vi "State Change Core.vi"(8 "error in":errorcluster, 10 "Transition State":refnum<class "State Pattern.lvclass">, 11 "State in":refnum<class "State Pattern.lvclass">) -> (0 "error out":errorcluster, 3 "State out":refnum<class "State Pattern.lvclass">)   [LabVIEW 2021, in "State Pattern.lvclass"]
uses:
  State Pattern.lvclass
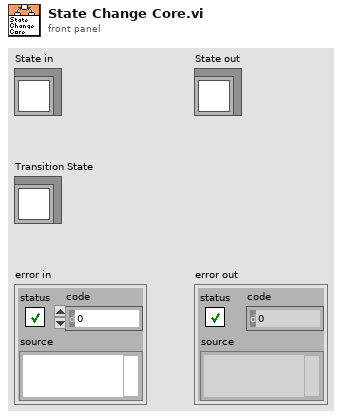
[diagram p1: front panel]
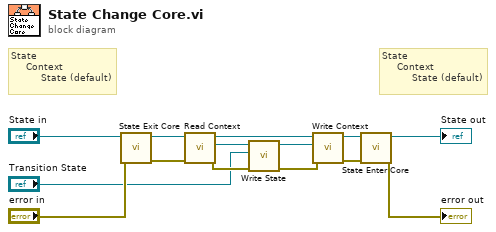
[diagram p0: block diagram]
diagram:
  # "State\n     Context\n          State (default)"
  # "State\n     Context\n          State (default)"
  n1 = call-dynamic "State Exit Core.vi"("error in"="error in", "State in"="State in") -> ("error out"=w5:errorcluster, "State out"=w10:refnum<class "State Pattern.lvclass">)  [unwired: 8 in]
  n2 = call-dynamic "Read Context.vi"("error in"=w5, "State in"=w10) -> ("error out"=w4:errorcluster, "Context"=w9:refnum<class "State Pattern.lvclass">, "State out"=w8:refnum<class "State Pattern.lvclass">)  [unwired: 7 in]
  n3 = call-dynamic "Write State.vi"("error in"=w4, "State"="Transition State", "Context in"=w9) -> ("error out"=w3:errorcluster, "Context out"=w6:refnum<class "State Pattern.lvclass">)  [unwired: 7 in]
  n4 = call-dynamic "Write Context.vi"("error in"=w3, "Context"=w6, "State in"=w8) -> ("error out"=w2:errorcluster, "State out"=w7:refnum<class "State Pattern.lvclass">)  [unwired: 7 in]
  n5 = call-dynamic "State Enter Core.vi"("error in"=w2, "State in"=w7) -> ("error out"=→"error out":errorcluster, "State out"=→"State out":refnum<class "State Pattern.lvclass">)  [unwired: 8 in]
